vi "WPI_SimpleGyro_Get Rate.vi"(8 "error in":errorcluster, 11 "SimpleGyroDevRef":T1) -> (0 "error out":errorcluster, 2 "Rate":dbl, 3 "SimpleGyroDevRef":T1)   [LabVIEW 2015, in "SimpleGyro.lvlib"]
uses:
  SimpleGyro.lvlib
  WPI_SimpleGyroDevRef.ctl
  <vilib>/Rock Robotics/SystemInterfaces/spilib/spi_bus.ctl
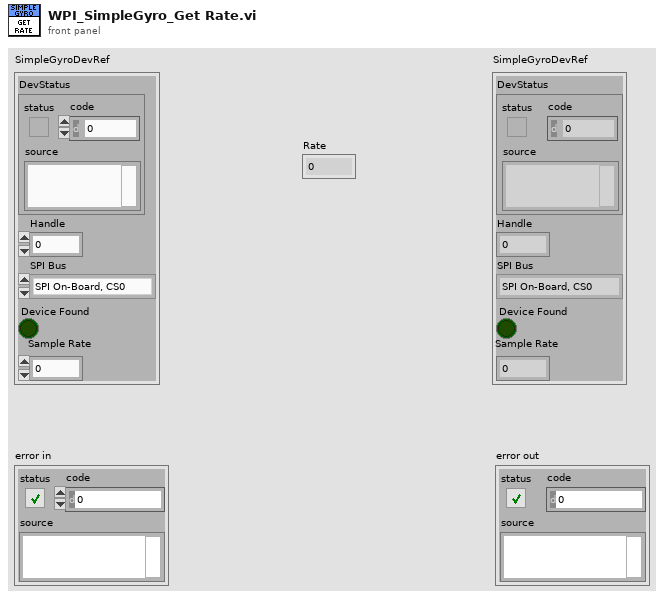
[diagram p1: front panel]
types:
  T1 = typedef "SimpleGyro.lvlib/WPI_SimpleGyroDevRef.ctl" = cluster{"DevStatus":errorcluster, "Handle":i32, "SPI Bus":T2, "Device Found":bool, "Sample Rate":dbl}
  T2 = typedef "spi_bus.ctl" = enum16{"SPI On-Board, CS0", "SPI On-Board, CS1", "SPI On-Board, CS2", "SPI On-Board, CS3", "SPI MXP", "Invalid"}
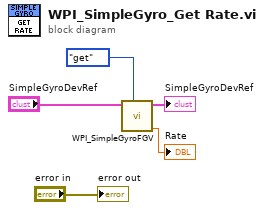
[diagram p0: block diagram]
diagram:
  n1 = call "WPI_SimpleGyroFGV.vi"("Operation"=enum16{"set", "get"}."get", "SimpleGyroDevRef"="SimpleGyroDevRef") -> ("Rate"=→"Rate":dbl, "SimpleGyroDevRef"=→"SimpleGyroDevRef":T1)  [unwired: 6 in, 2 out]
  "error out" <- "error in"
